vi "setStateChangedEvent.vi"(10 "StateChangedEvent":refnum<user-event>, 11 "UserEvents in":refnum<class "UserEvents.lvclass">) -> (3 "UserEvents out":refnum<class "UserEvents.lvclass">)   [LabVIEW 2016, in "UserEvents.lvclass"]
uses:
  UserEvents.lvclass
  Types/StateChangedEvent.ctl
  Types/Timestamp.ctl
  Types/SummaryStates.ctl
  Types/DetailedStates.ctl
  UserEvents.lvclass/UserEvents.ctl
  Types/M1M3SupportTypes.lvlib
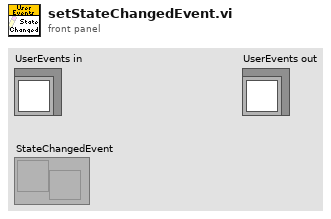
[diagram p1: front panel]
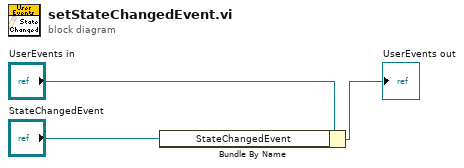
[diagram p0: block diagram]
diagram:
  n1 = Bundle By Name(cluster="UserEvents in", "StateChangedEvent"="StateChangedEvent") -> (→"UserEvents out":refnum<class "UserEvents.lvclass">)
